vi "PixieGetDataold.vi"(8 "error IO":errorcluster) -> (0 "error out":errorcluster, 1 "Run time [s]":dbl, 2 "CH1 LT":dbl, 3 "CH0 LT":dbl, 4 "CH1 SFDT":dbl, 5 "Histogram Data":u32[][](array[numeric]), 6 "CH0 SFDT":dbl, 7 "CH1 GDT":dbl, 11 "CH0 GDT":dbl)   [LabVIEW 2011]
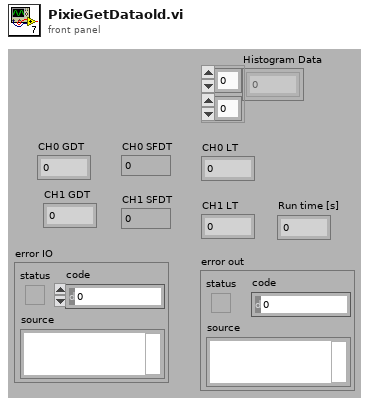
[diagram p1: front panel]
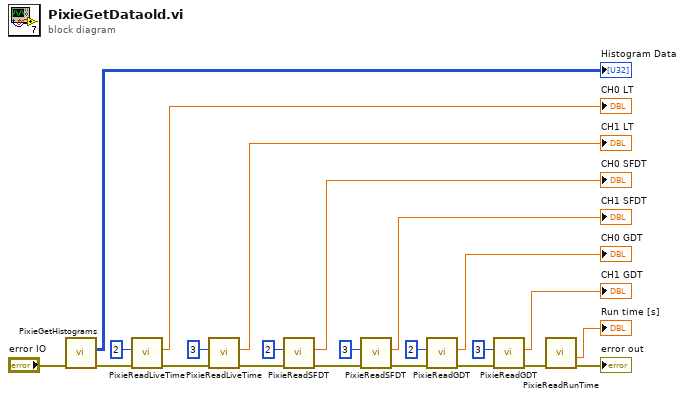
[diagram p0: block diagram]
diagram:
  n1 = call "PixieGetHistograms.vi"("error in (no error)"="error IO") -> ("error out"=w18:errorcluster, "Histogram Data"=→"Histogram Data":u32[][])  [unwired: 1 in, 8 out]
  n2 = call "PixieReadLiveTime.vi"("error in (no error)"=w18, "ChanNum"=u16 2) -> ("error out"=w17:errorcluster, "livetime"=→"CH0 LT":dbl)  [unwired: 8 out]
  n3 = call "PixieReadLiveTime.vi"("error in (no error)"=w17, "ChanNum"=u16 3) -> ("error out"=w13:errorcluster, "livetime"=→"CH1 LT":dbl)  [unwired: 8 out]
  n4 = call "PixieReadSFDT.vi"("error in (no error)"=w13, "ChanNum"=u16 2) -> ("error out"=w8:errorcluster, "SFDT"=→"CH0 SFDT":dbl)  [unwired: 8 in]
  n5 = call "PixieReadSFDT.vi"("error in (no error)"=w8, "ChanNum"=u16 3) -> ("error out"=w4:errorcluster, "SFDT"=→"CH1 SFDT":dbl)  [unwired: 8 in]
  n6 = call "PixieReadGDT.vi"("error in (no error)"=w4, "ChanNum"=u16 2) -> ("error out"=w5:errorcluster, "GDT"=→"CH0 GDT":dbl)  [unwired: 8 in]
  n7 = call "PixieReadGDT.vi"("error in (no error)"=w5, "ChanNum"=u16 3) -> ("error out"=w3:errorcluster, "GDT"=→"CH1 GDT":dbl)  [unwired: 8 in]
  n8 = call "PixieReadRunTime.vi"("error in (no error)"=w3) -> ("error out"=→"error out":errorcluster, "Run time [s]"=→"Run time [s]":dbl)  [unwired: 1 in, 8 out]
